vi "SET_Build Language List.vi"() -> ()   [LabVIEW 2013]
panel:
  in  "file (use dialog)":path
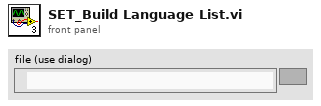
[diagram p1: front panel]
types:
  T1 = cluster{"Name":string, "Tag":string, "Code Page":u16}[]
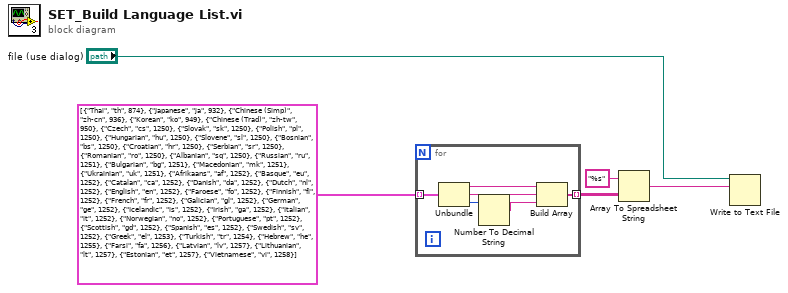
[diagram p0: block diagram]
diagram:
  n1 = for {
    tunnel: T1 [{"Name"="Thai", "Tag"="th", "Code Page"=874}, {"Name"="Japanese", "Tag"="ja", "Code Page"=932}, {"Name"="Chinese (Simp)", "Tag"="zh-cn", "Code Page"=936}, {"Name"="Korean", "Tag"="ko", "Code Page"=949}, {"Name"="Chinese (Trad)", "Tag"="zh-tw", "Code Page"=950}, {"Name"="Czech", "Tag"="cs", "Code Page"=1250}, {"Name"="Slovak", "Tag"="sk", "Code Page"=1250}, {"Name"="Polish", "Tag"="pl", "Code Page"=1250}, {"Name"="Hungarian", "Tag"="hu", "Code Page"=1250}, {"Name"="Slovene", "Tag"="sl", "Code Page"=1250}, {"Name"="Bosnian", "Tag"="bs", "Code Page"=1250}, {"Name"="Croatian", "Tag"="hr", "Code Page"=1250}, {"Name"="Serbian", "Tag"="sr", "Code Page"=1250}, {"Name"="Romanian", "Tag"="ro", "Code Page"=1250}, {"Name"="Albanian", "Tag"="sq", "Code Page"=1250}, {"Name"="Russian", "Tag"="ru", "Code Page"=1251}, {"Name"="Bulgarian", "Tag"="bg", "Code Page"=1251}, {"Name"="Macedonian", "Tag"="mk", "Code Page"=1251}, {"Name"="Ukrainian", "Tag"="uk", "Code Page"=1251}, {"Name"="Afrikaans", "Tag"="af", "Code Page"=1252}, {"Name"="Basque", "Tag"="eu", "Code Page"=1252}, {"Name"="Catalan", "Tag"="ca", "Code Page"=1252}, {"Name"="Danish", "Tag"="da", "Code Page"=1252}, {"Name"="Dutch", "Tag"="nl", "Code Page"=1252}, {"Name"="English", "Tag"="en", "Code Page"=1252}, {"Name"="Faroese", "Tag"="fo", "Code Page"=1252}, {"Name"="Finnish", "Tag"="fi", "Code Page"=1252}, {"Name"="French", "Tag"="fr", "Code Page"=1252}, {"Name"="Galician", "Tag"="gl", "Code Page"=1252}, {"Name"="German", "Tag"="ge", "Code Page"=1252}, {"Name"="Icelandic", "Tag"="is", "Code Page"=1252}, {"Name"="Irish", "Tag"="ga", "Code Page"=1252}, {"Name"="Italian", "Tag"="it", "Code Page"=1252}, {"Name"="Norwegian", "Tag"="no", "Code Page"=1252}, {"Name"="Portuguese", "Tag"="pt", "Code Page"=1252}, {"Name"="Scottish", "Tag"="gd", "Code Page"=1252}, {"Name"="Spanish", "Tag"="es", "Code Page"=1252}, {"Name"="Swedish", "Tag"="sv", "Code Page"=1252}, {"Name"="Greek", "Tag"="el", "Code Page"=1253}, {"Name"="Turkish", "Tag"="tr", "Code Page"=1254}, {"Name"="Hebrew", "Tag"="he", "Code Page"=1255}, {"Name"="Farsi", "Tag"="fa", "Code Page"=1256}, {"Name"="Latvian", "Tag"="lv", "Code Page"=1257}, {"Name"="Lithuanian", "Tag"="lt", "Code Page"=1257}, {"Name"="Estonian", "Tag"="et", "Code Page"=1257}, {"Name"="Vietnamese", "Tag"="vi", "Code Page"=1258}] -> [w11] mode=indexing
    tunnel: [w6] -> w4 mode=indexing
    n2 = Unbundle(w11) -> ("Name"=w9:string, "Tag"=w8:string, "Code Page"=w10:u16)
    n3 = Number To Decimal String(number=w10) -> (decimal integer string=w7:string)  [unwired: 1 in]
    n4 = Build Array(w9, w8, w7) -> (w6:string[])
  }
  n5 = Array To Spreadsheet String(array=w4, 3:"%s" ("format string")) -> (spreadsheet string=w2:string)  [unwired: 1 in]
  n6 = Write to Text File(file (use dialog)="file (use dialog)", text=w2) -> ()  [unwired: 2 in, 3 out]
